vi "Subvi detector.vi"(10 "Memory label":refnum<k21>="CI01 buffer", 11 "DI channel":refnum<k21>="Connector0/DIO1") -> ()   [LabVIEW 2017]
uses:
  <vilib>/Platform/TimedLoop/XDataNode/timing_clust.ctl
  <vilib>/Platform/TimedLoop/XDataNode/nitl_modes.ctl
  <vilib>/Platform/TimedLoop/XDataNode/wakeup.ctl
  <vilib>/rvi/Emulation/niFpgaSctlEmulationGetInTimedLoop.vi
  <vilib>/rvi/Emulation/niFpgaEmulationReportErrorSimple.vi
  <vilib>/rvi/Emulation/niFpgaGetClockAttributes.vi
  <vilib>/rvi/Emulation/niFpgaCriticalErrorInLSC.vi
  <vilib>/rvi/Emulation/niFpgaProcessEmulError.vi
  GV pixel clock count.vi
  GV line gating.vi
  <vilib>/rvi/eio/common/nirviEmuTemplateMethod_errors.vi
  <vilib>/Platform/TimedLoop/XDataNode/XDataNode.xnode
  <vilib>/eio/EIONode/EIONode.xnode
  <vilib>/Platform/TimedLoop/XDataNode/XDNodeRunTimeDep.lvlib
  Probes/GV DO4.vi
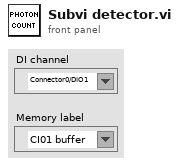
[diagram p1: front panel]
types:
  T1 = typedef "XDNodeRunTimeDep.lvlib/timing_clust.ctl" = cluster{"Expected End [f-1]":u64, "Actual End [f-1]":u64, "Finished Late? [f-1]":bool, "Expected End [i-1]":u64, "Actual End [i-1]":u64, "Finished Late? [i-1]":bool, "Expected Start [i]":u64, "Actual Start [i]":u64, "Expected Start [f]":u64, "Actual Start [f]":u64, "Source Name":string, "Structure Name":string, "Period":i64, "Deadline":i64, "Offset":i64, "Start":i64, "Priority":i32, "Timeout":i32, "Mode":T2, "Wakeup Reason":T3, "Error":errorcluster, "Source Type":string, "Secondary Source Type":string, "Global End Time":u64, "Global Start Time":u64, "Frame Duration":u64, "Iteration Duration":u64, "Assigned CPU":i32, "I/O Scan Engine Mode":u32}
  T2 = typedef "XDNodeRunTimeDep.lvlib/nitl_modes.ctl" = enum32{"No Change", "Process missed periods, maintain original phase", "Discard missed periods, maintain original phase", "Process missed periods, ignore original phase", "Discard missed periods, ignore original phase"}
  T3 = typedef "XDNodeRunTimeDep.lvlib/wakeup.ctl" = enum32{"Normal", "Aborted", "Asynchronous wakeup", "Timing source error", "Timed loop error", "Timeout"}
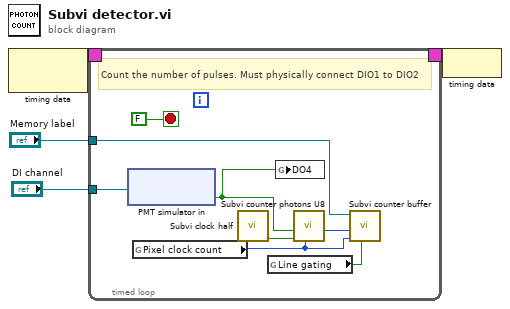
[diagram p0: block diagram]
diagram:
  n1 = node-c288() -> (w4:T1)  [unwired: 1 in]
  n2 = timed-loop {
    timing: w4 -> [_]
    timing-out: [_] -> w3
    tunnel: "Memory label" -> [w12]
    tunnel: "DI channel" -> [w9]
    stop <- FALSE stop-if-true
    # "Count the number of pulses. Must physically connect DIO1 to DIO2"
    n3 = xnode "PMT simulator in"("FPGA I/O In"=w9) -> ("I/O Item"=w5:bool)  [unwired: 1 out]
    n4 = global read "GV pixel clock count.vi" "Pixel clock count"() -> (w8:u16)
    n5 = call "Subvi clock half.vi"() -> ("Output"=w11:bool)  [unwired: 11 in]
    n6 = global read "GV line gating.vi" "Line gating"() -> (w6:bool)
    n7 = global write "GV DO4.vi" "DO4"(w5) -> ()
    n8 = call "Subvi counter photons U8.vi"("Pixel clock"=w8, "Clock"=w11, "Single photon"=w5) -> ("Photon count"=w7:u8)  [unwired: 8 in]
    n9 = call "Subvi counter buffer.vi"("Line gating"=w6, "Pixel count"=w8, "Photon count"=w7, "Memory In"=w12) -> ()  [unwired: 8 in]
  }
  n10 = node-c288(w3) -> ()
